vi "read.vi"   [LabVIEW 2012]
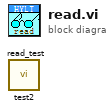
[diagram p0: block diagram]
diagram:
  n1 = call "test2.vi"() -> ()  [unwired: 9 in, 3 out]
  n2 = call "read_test.vi"() -> ()  [unwired: 9 in, 3 out]
